vi "Add Member Data.vi"(8 "error in (no error)":errorcluster, 11 "Message Scripter in":refnum<class "Message Scripter.lvclass">) -> (0 "error out":errorcluster, 3 "Message Scripter out":refnum<class "Message Scripter.lvclass">)   [LabVIEW 2020, in "Message Maker.lvlib" / "Message Scripter.lvclass"]
uses:
  Message Scripter.lvclass
  Message Maker.lvlib
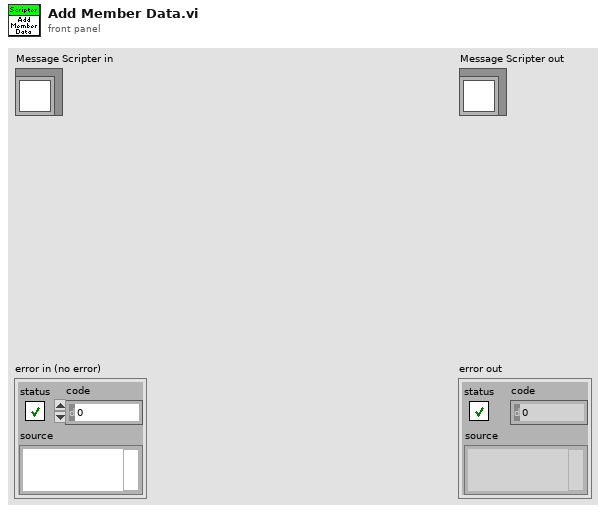
[diagram p1: front panel]
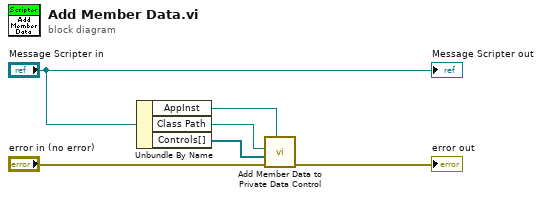
[diagram p0: block diagram]
diagram:
  n1 = Unbundle By Name("Message Scripter in") -> ("AppInst"=w6:refnum<vi>, "Class Path"=w5:path, "Controls[]"=w2:refnum<vi>[])
  n2 = call "Add Member Data to Private Data Control.vi"("AppInst"=w6, "error in (no error)"="error in (no error)", "Controls"=w2, "Target Path"=w5) -> ("error out"=→"error out":errorcluster)  [unwired: 7 in]
  "Message Scripter out" <- "Message Scripter in"
